vi "FFT Power Spectral Density for N Chan (CDB).vi"(6 "averaging parameters":T1={"averaging mode"=enum."No averaging", "weighting mode"=enum."Exponential", "number of averages"=10} {"number of averages" min=1}, 7 "restart averaging (F)":bool, 8 "error in (no error)":errorcluster, 9 "dB On (F)":bool, 10 "window":T2=1 items=["Rectangle"=0, "Hanning"=1, "Hamming"=2, "Blackman-Harris"=3, "Exact Blackman"=4, "Blackman"=5, "Flat Top"=6, "4 Term B-Harris "=7, "7 Term B-Harris"=8, "Low Sidelobe"=9, "Blackman Nuttall"=11, "Triangle"=30, "Bartlett-Hanning"=31, "Bohman"=32, "Parzen"=33, "Welch"=34, "Kaiser"=60, "Dolph-Chebyshev"=61, "Gaussian"=62], 11 "time signals":waveform(cdb)[](array[waveform])) -> (0 "error out":errorcluster, 1 "averages completed":dbl, 3 "power spectral densities":cluster{"f0":dbl, "df":dbl, "magnitude":dbl[]}[](array[cluster]) {"magnitude" format="%.2p"; "f0" format="%.2p"; "df" format="%.2p"}, 5 "averaging done":bool)   [LabVIEW 2020, in "NI_MAPro.lvlib"]
doc: "Computes the averaged power spectral density of <B>time signal</B>. You can use this polymorphic VI to compute the averaged power spectral density of a single channel or multiple channel signal. The data type you wire to the <B>time signal</B> input determines the polymorphic instance to use."
uses:
  NI_MAPro.lvlib
  windowTd.ctl
  NI_MABase.lvlib
  NI_AALPro.lvlib
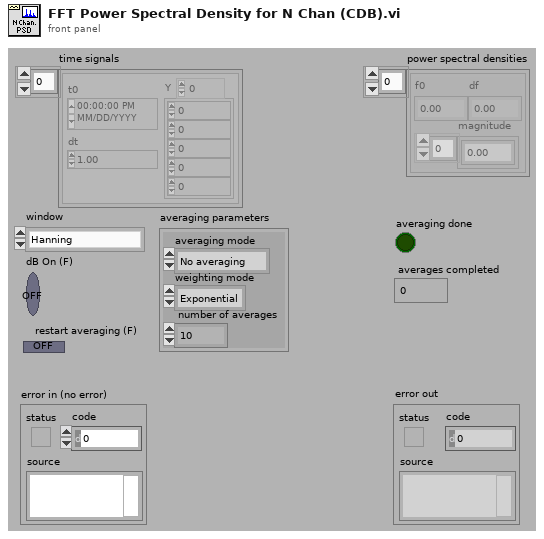
[diagram p1: front panel]
types:
  T1 = cluster{"averaging mode":enum16{"No averaging", "Vector averaging", "RMS averaging", "Peak hold"}, "weighting mode":enum16{"Linear", "Exponential"}, "number of averages":u32}
  T2 = typedef "NI_AALPro.lvlib/windowTd.ctl" = u32
  T3 = cluster{"block size":i32, "dt":dbl, "spectrum parameters":cluster{"averaging parameters":cluster{"averaging mode":enum16{"No averaging", "Vector averaging", "RMS averaging", "Peak hold"}, "weighting mode":enum16{"Linear", "Exponential"}, "number of averages":u32}, "window":T2}, "df":dbl, "averages completed":dbl, "complex spectrum":cdb[], "real spectrum":dbl[], "t0 history":dbl, "dt history":dbl, "timestamp":dbl, "lin avg done":bool}
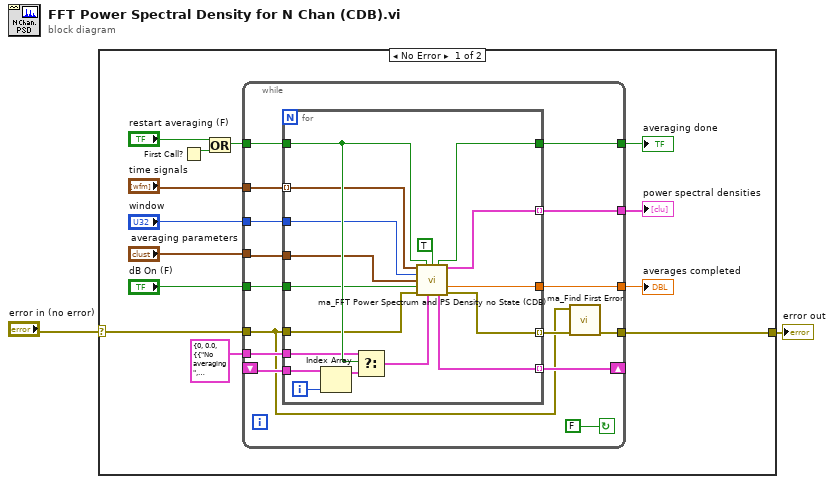
[diagram p0: block diagram]
diagram:
  n1 = case shown="No Error" "error in (no error)" {
    selector: "error in (no error)" -> [w4 w48]
    tunnel: [w5 w48] -> w2
    frame No Error {
      n2 = First Call?() -> (First Call?: T/F=w14:bool)
      n3 = Or(x="restart averaging (F)", y=w14) -> (x .or. y?=w13:bool)
      n4 = while {
        tunnel: "window" -> [w21]
        tunnel: w4 -> [w16]
        tunnel: "time signals" -> [w20]
        tunnel: "averaging parameters" -> [w19]
        tunnel: w13 -> [w25]
        tunnel: [w30] -> w8
        tunnel: [w29] -> w6
        tunnel: [w28] -> w7
        tunnel: [w17] -> w5
        shift-right: [w26] -> _
        shift-left: _ -> [w24]
        tunnel: T3 {"block size"=0, "dt"=0.0, "spectrum parameters"={"averaging parameters"={"averaging mode"=enum."No averaging", "weighting mode"=enum."Linear", "number of averages"=0}, "window"=0}, "df"=0.0, "averages completed"=0.0, "complex spectrum"=[], "real spectrum"=[], "t0 history"=0.0, "dt history"=0.0, "timestamp"=0.0, "lin avg done"=FALSE} ("state info") -> [w23]
        tunnel: "dB On (F)" -> [w22]
        stop <- FALSE continue-if-true
        n5 = for {
          tunnel: [w47] -> w30
          tunnel: [w46] -> w29
          tunnel: [w45] -> w28 mode=indexing
          tunnel: [w44] -> w27 mode=indexing
          tunnel: [w43] -> w26 mode=indexing
          tunnel: w25 -> [w42]
          tunnel: w24 -> [w34]
          tunnel: w23 -> [w40]
          tunnel: w16 -> [w39]
          tunnel: w22 -> [w38]
          tunnel: w21 -> [w37]
          tunnel: w20 -> [w36] mode=indexing
          tunnel: w19 -> [w35]
          i -> [w33]
          n6 = Index Array(array=w34, index=w33) -> (element=w32:T3)
          n7 = Select(t=w40, s=w42, f=w32) -> (s? t:f=w41:T3)
          n8 = call "ma_FFT Power Spectrum and PS Density no State (CDB).vi"("time signal"=w36, "restart averaging (F)"=w42, "ps density"=TRUE, "window"=w37, "averaging parameters"=w35, "dB On (F)"=w38, "error in"=w39, "state info"=w41) -> ("averaging done"=w47:bool, "power spectrum"=w45:cluster{"f0":dbl, "df":dbl, "magnitude":dbl[]}, "averages completed"=w46:dbl, "state info"=w43:T3, "error out"=w44:errorcluster)  [unwired: 1 in, 2 out]
        }
        n9 = call "ma_Find First Error.vi"("error array in"=w27, "error in 1 (no error)"=w16) -> ("error out"=w17:errorcluster)  [unwired: 2 in, 3 out]
      }
      "averaging done" <- w8
      "averages completed" <- w6
      "power spectral densities" <- w7
    }
    frame Error {
    }
  }
  "error out" <- w2
